vi "加载所有配置.vi"(1 "error in (no error)":errorcluster caption="错误输入（无错误）") -> (0 "error out":errorcluster caption="错误输出")   [LabVIEW 2014]
doc: "该模板用于创建子VI。"
uses:
  glb/glb_data.vi
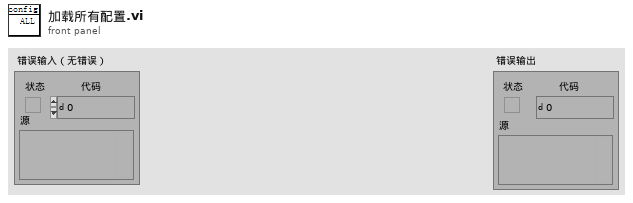
[diagram p1: front panel]
types:
  T1 = cluster{"名称":string, "简称":string, "单位":string, "附加":string[], "类型":enum16{"测试模块", "FPGA", "cRIO", "其他设备", "总体展示"}}[]
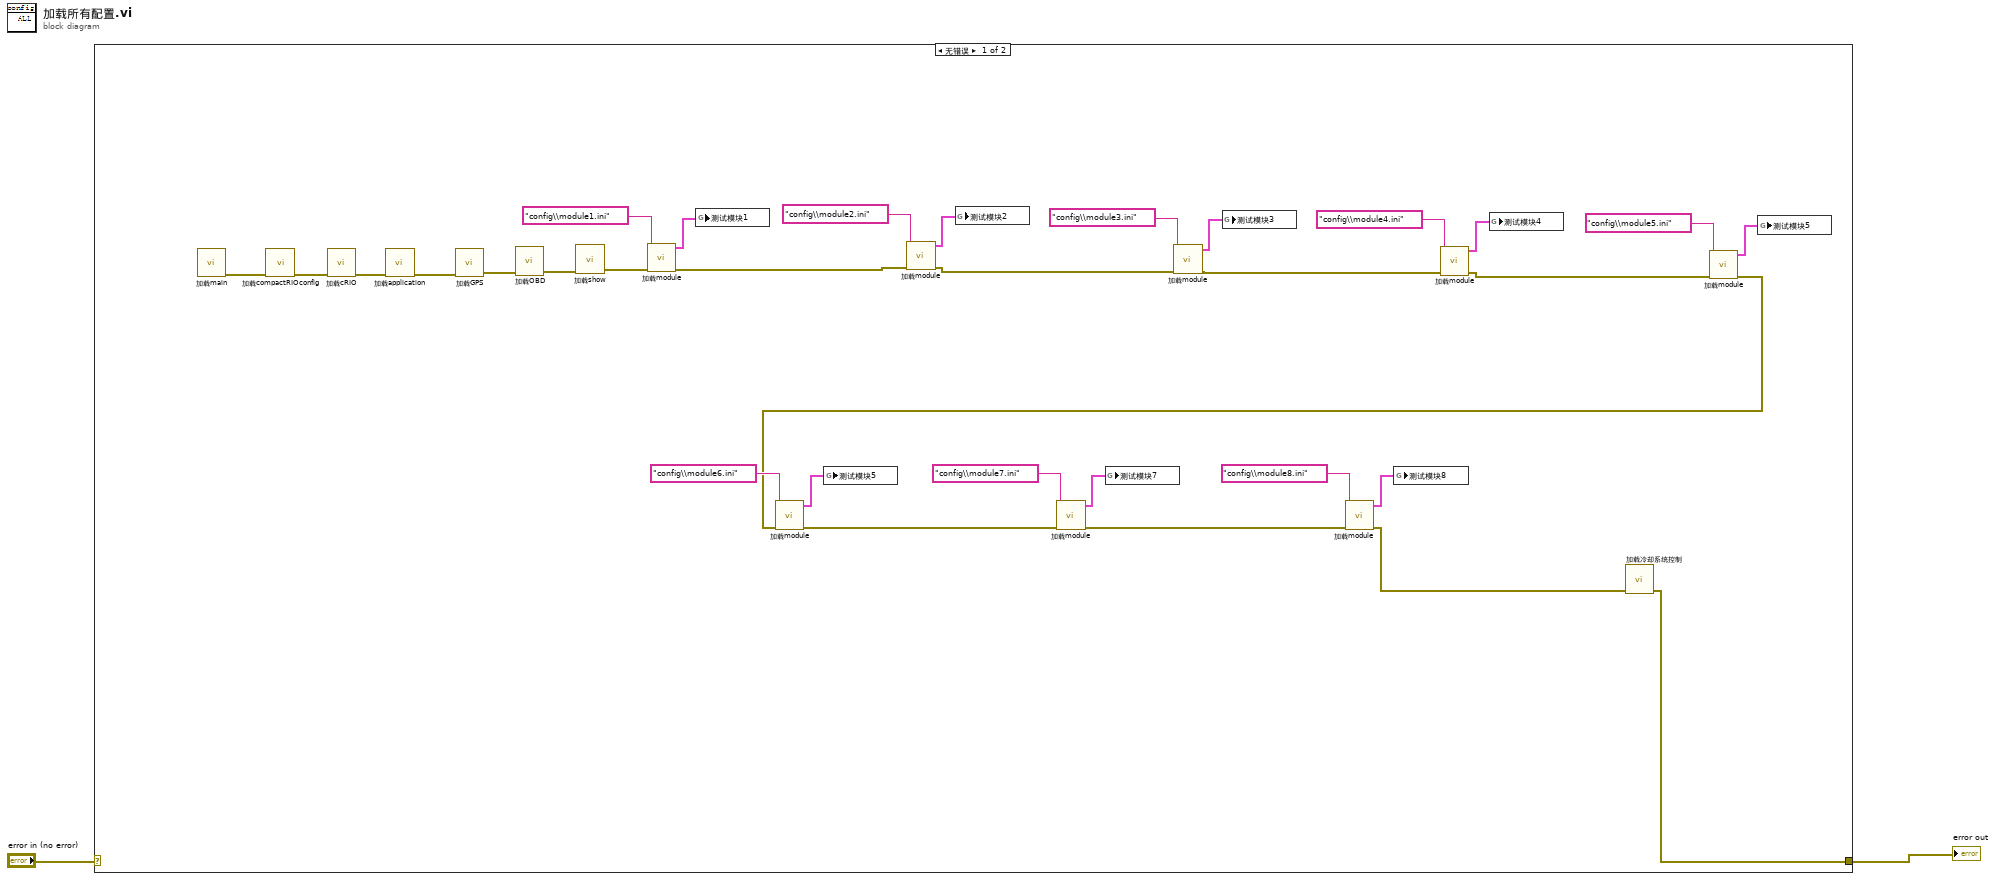
[diagram p0: block diagram]
diagram:
  n1 = case shown="无错误" "error in (no error)" {
    selector: "error in (no error)" -> [_ w35]
    tunnel: [w3 w35] -> w1
    frame No Error {
      n2 = call "加载main.vi"() -> ("error out"=w5:errorcluster)  [unwired: 11 in]
      n3 = call "加载compactRIOconfig.vi"("error in (no error)"=w5) -> ("error out"=w6:errorcluster)  [unwired: 10 in]
      n4 = call "加载cRIO.vi"("error in (no error)"=w6) -> ("error out"=w7:errorcluster)  [unwired: 10 in]
      n5 = call "加载application.vi"("error in (no error)"=w7) -> ("error out"=w34:errorcluster)  [unwired: 10 in]
      n6 = call "加载GPS.vi"("error in (no error)"=w34) -> ("error out"=w33:errorcluster)  [unwired: 10 in]
      n7 = call "加载OBD.vi"("error in (no error)"=w33) -> ("error out"=w32:errorcluster)  [unwired: 10 in]
      n8 = call "加载show.vi"("error in (no error)"=w32) -> ("error out"=w31:errorcluster)  [unwired: 10 in]
      n9 = call "加载module.vi"("error in (no error)"=w31, "测试模块配置文件"="config\\module1.ini") -> ("error out"=w14:errorcluster, "测试模块配置文件输出"=w29:T1)  [unwired: 8 in]
      n10 = global write "glb_data.vi" "测试模块1"(w29) -> ()
      n11 = call "加载module.vi"("error in (no error)"=w14, "测试模块配置文件"="config\\module2.ini") -> ("error out"=w13:errorcluster, "测试模块配置文件输出"=w28:T1)  [unwired: 8 in]
      n12 = global write "glb_data.vi" "测试模块2"(w28) -> ()
      n13 = call "加载module.vi"("error in (no error)"=w13, "测试模块配置文件"="config\\module3.ini") -> ("error out"=w12:errorcluster, "测试模块配置文件输出"=w25:T1)  [unwired: 8 in]
      n14 = global write "glb_data.vi" "测试模块3"(w25) -> ()
      n15 = call "加载module.vi"("error in (no error)"=w12, "测试模块配置文件"="config\\module4.ini") -> ("error out"=w11:errorcluster, "测试模块配置文件输出"=w24:T1)  [unwired: 8 in]
      n16 = global write "glb_data.vi" "测试模块4"(w24) -> ()
      n17 = call "加载module.vi"("error in (no error)"=w11, "测试模块配置文件"="config\\module5.ini") -> ("error out"=w10:errorcluster, "测试模块配置文件输出"=w21:T1)  [unwired: 8 in]
      n18 = call "加载module.vi"("error in (no error)"=w10, "测试模块配置文件"="config\\module6.ini") -> ("error out"=w9:errorcluster, "测试模块配置文件输出"=w20:T1)  [unwired: 8 in]
      n19 = global write "glb_data.vi" "测试模块5"(w20) -> ()
      n20 = call "加载module.vi"("error in (no error)"=w9, "测试模块配置文件"="config\\module7.ini") -> ("error out"=w8:errorcluster, "测试模块配置文件输出"=w17:T1)  [unwired: 8 in]
      n21 = global write "glb_data.vi" "测试模块7"(w17) -> ()
      n22 = call "加载module.vi"("error in (no error)"=w8, "测试模块配置文件"="config\\module8.ini") -> ("error out"=w4:errorcluster, "测试模块配置文件输出"=w16:T1)  [unwired: 8 in]
      n23 = global write "glb_data.vi" "测试模块8"(w16) -> ()
      n24 = call "加载冷却系统控制.vi"("error in (no error)"=w4) -> ("error out"=w3:errorcluster)  [unwired: 10 in]
      n25 = global write "glb_data.vi" "测试模块5"(w21) -> ()
    }
    frame Error {
    }
  }
  "error out" <- w1
